vi "DisplayJson.vi"(11 "JSON String In":string="[{\"version\":\"1.0.0\",\"header\":{\"creationDate\":\"2022-06-03T00:00:00\",\"remarks\":\"\",\"serialNumber\":\"98172\",\"productNumber\":\"123021.1804\",\"productType\":\"PAA-9L\",\"pressureType\":2,\"productSeries\":\"9L\",\"compensatedTemperatureRange\":{\"min\":-10.0,\"max\":80.0,\"unit\":4},\"compensatedPressureRange\":{\"min\":0.0,\"max\":0.35,\"unit\":3},\"electricSupply\":{\"magnitude\":1.0,\"unit\":18},\"orderNumber\":9990266,\"orderPosition\":3,\"orderTargetDispatchDate\":\"2022-06-02T00:00:00+00:00\",\"customerName\":\"DemoData Inc.\",\"customerNumber\":12345678,\"customerOrderNumber\":\"Cust-9990266-123\",\"customerReferenceNumber\":\"\",\"customerProductT...") -> ()   [LabVIEW 2017] (continued)
\"unit\":4}}}}}},{\"reference\":\"F_12300_XX_0000098765\",\"environmentTarget\":{\"pressure\":{\"magnitude\":0.11,\"unit\":3},\"temperature\":{\"magnitude\":40.0,\"unit\":4}},\"environment\":{\"pressure\":{\"magnitude\":0.110005,\"unit\":3},\"temperature\":{\"magnitude\":39.7284,\"unit\":4},\"supply\":{\"magnitude\":1.0,\"unit\":18}},\"raw\":{\"signal\":{\"magnitude\":28.847389263,\"unit\":22},\"bridgeResistance\":{\"magnitude\":3661.6768749,\"unit\":28}},\"compensated\":{\"mathematicalModels\":{\"MM0123\":{\"pressure\":{\"output\":{\"magnitude\":0.109977,\"unit\":3},\"error\":{\"magnitude\":-0.0080257298,\"unit\":7}},\"temperature\":{\"output\":{\"magnitude\":39.719,\"unit\":4},\"error\":{\"magnitude\":-0.0094531335,\"unit\":4}}}}}},{\"reference\":\"F_12300_XX_0000098765\",\"environmentTarget\":{\"pressure\":{\"magnitude\":0.19,\"unit\":3},\"temperature\":{\"magnitude\":40.0,\"unit\":4}},\"environment\":{\"pressure\":{\"magnitude\":0.190007,\"unit\":3},\"temperature\":{\"magnitude\":39.7284,\"unit\":4},\"supply\":{\"magnitude\":1.0,\"unit\":18}},\"raw\":{\"signal\":{\"magnitude\":40.361547993,\"unit\":22},\"bridgeResistance\":{\"magnitude\":3657.3317258,\"unit\":28}},\"compensated\":{\"mathematicalModels\":{\"MM0123\":{\"pressure\":{\"output\":{\"magnitude\":0.190005,\"unit\":3},\"error\":{\"magnitude\":-0.00061989229,\"unit\":7}},\"temperature\":{\"output\":{\"magnitude\":39.7158,\"unit\":4},\"error\":{\"magnitude\":-0.012650311,\"unit\":4}}}}}},{\"reference\":\"F_12300_XX_0000098765\",\"environmentTarget\":{\"pressure\":{\"magnitude\":0.27,\"unit\":3},\"temperature\":{\"magnitude\":40.0,\"unit\":4}},\"environment\":{\"pressure\":{\"magnitude\":0.269994,\"unit\":3},\"temperature\":{\"magnitude\":39.7284,\"unit\":4},\"supply\":{\"magnitude\":1.0,\"unit\":18}},\"raw\":{\"signal\":{\"magnitude\":51.835430308,\"unit\":22},\"bridgeResistance\":{\"magnitude\":3653.059498,\"unit\":28}},\"compensated\":{\"mathematicalModels\":{\"MM0123\":{\"pressure\":{\"output\":{\"magnitude\":0.270012,\"unit\":3},\"error\":{\"magnitude\":0.0052035531,\"unit\":7}},\"temperature\":{\"output\":{\"magnitude\":39.7125,\"unit\":4},\"error\":{\"magnitude\":-0.015896776,\"unit\":4}}}}}},{\"reference\":\"F_12300_XX_0000098765\",\"environmentTarget\":{\"pressure\":{\"magnitude\":0.35,\"unit\":3},\"temperature\":{\"magnitude\":40.0,\"unit\":4}},\"environment\":{\"pressure\":{\"magnitude\":0.350005,\"unit\":3},\"temperature\":{\"magnitude\":39.7284,\"unit\":4},\"supply\":{\"magnitude\":1.0,\"unit\":18}},\"raw\":{\"signal\":{\"magnitude\":63.26645716,\"unit\":22},\"bridgeResistance\":{\"magnitude\":3648.8999829,\"unit\":28}},\"compensated\":{\"mathematicalModels\":{\"MM0123\":{\"pressure\":{\"output\":{\"magnitude\":0.349978,\"unit\":3},\"error\":{\"magnitude\":-0.0076198189,\"unit\":7}},\"temperature\":{\"output\":{\"magnitude\":39.7135,\"unit\":4},\"error\":{\"magnitude\":-0.014908129,\"unit\":4}}}}}},{\"reference\":\"F_12300_XX_0000098765\",\"environmentTarget\":{\"pressure\":{\"magnitude\":0.03,\"unit\":3},\"temperature\":{\"magnitude\":60.0,\"unit\":4}},\"environment\":{\"pressure\":{\"magnitude\":0.029994,\"unit\":3},\"temperature\":{\"magnitude\":59.8651,\"unit\":4},\"supply\":{\"magnitude\":1.0,\"unit\":18}},\"raw\":{\"signal\":{\"magnitude\":18.423541771,\"unit\":22},\"bridgeResistance\":{\"magnitude\":3857.3811421,\"unit\":28}},\"compensated\":{\"mathematicalModels\":{\"MM0123\":{\"pressure\":{\"output\":{\"magnitude\":0.0300054,\"unit\":3},\"error\":{\"magnitude\":0.0032489215,\"unit\":7}},\"temperature\":{\"output\":{\"magnitude\":59.9297,\"unit\":4},\"error\":{\"magnitude\":0.064540842,\"unit\":4}}}}}},{\"reference\":\"F_12300_XX_0000098765\",\"environmentTarget\":{\"pressure\":{\"magnitude\":0.11,\"unit\":3},\"temperature\":{\"magnitude\":60.0,\"unit\":4}},\"environment\":{\"pressure\":{\"magnitude\":0.110001,\"unit\":3},\"temperature\":{\"magnitude\":59.8651,\"unit\":4},\"supply\":{\"magnitude\":1.0,\"unit\":18}},\"raw\":{\"signal\":{\"magnitude\":30.058054899,\"unit\":22},\"bridgeResistance\":{\"magnitude\":3852.9241805,\"unit\":28}},\"compensated\":{\"mathematicalModels\":{\"MM0123\":{\"pressure\":{\"output\":{\"magnitude\":0.109972,\"unit\":3},\"error\":{\"magnitude\":-0.0083184018,\"unit\":7}},\"temperature\":{\"output\":{\"magnitude\":59.9321,\"unit\":4},\"error\":{\"magnitude\":0.066957365,\"unit\":4}}}}}},{\"reference\":\"F_12300_XX_0000098765\",\"environmentTarget\":{\"pressure\":{\"magnitude\":0.19,\"unit\":3},\"temperature\":{\"magnitude\":60.0,\"unit\":4}},\"environment\":{\"pressure\":{\"magnitude\":0.189998,\"unit\":3},\"temperature\":{\"magnitude\":59.8651,\"unit\":4},\"supply\":{\"magnitude\":1.0,\"unit\":18}},\"raw\":{\"signal\":{\"magnitude\":41.669413946,\"unit\":22},\"bridgeResistance\":{\"magnitude\":3848.535791,\"unit\":28}},\"compensated\":{\"mathematicalModels\":{\"MM0123\":{\"pressure\":{\"output\":{\"magnitude\":0.190007,\"unit\":3},\"error\":{\"magnitude\":0.0026498924,\"unit\":7}},\"temperature\":{\"output\":{\"magnitude\":59.9347,\"unit\":4},\"error\":{\"magnitude\":0.069571324,\"unit\":4}}}}}},{\"reference\":\"F_12300_XX_0000098765\",\"environmentTarget\":{\"pressure\":{\"magnitude\":0.27,\"unit\":3},\"temperature\":{\"magnitude\":60.0,\"unit\":4}},\"environment\":{\"pressure\":{\"magnitude\":0.270009,\"unit\":3},\"temperature\":{\"magnitude\":59.8651,\"unit\":4},\"supply\":{\"magnitude\":1.0,\"unit\":18}},\"raw\":{\"signal\":{\"magnitude\":53.245645567,\"unit\":22},\"bridgeResistance\":{\"magnitude\":3844.1953821,\"unit\":28}},\"compensated\":{\"mathematicalModels\":{\"MM0123\":{\"pressure\":{\"output\":{\"magnitude\":0.27003,\"unit\":3},\"error\":{\"magnitude\":0.0061415459,\"unit\":7}},\"temperature\":{\"output\":{\"magnitude\":59.935,\"unit\":4},\"error\":{\"magnitude\":0.069824739,\"unit\":4}}}}}},{\"reference\":\"F_12300_XX_0000098765\",\"environmentTarget\":{\"pressure\":{\"magnitude\":0.35,\"unit\":3},\"temperature\":{\"magnitude\":60.0,\"unit\":4}},\"environment\":{\"pressure\":{\"magnitude\":0.349993,\"unit\":3},\"temperature\":{\"magnitude\":59.8651,\"unit\":4},\"supply\":{\"magnitude\":1.0,\"unit\":18}},\"raw\":{\"signal\":{\"magnitude\":64.779425416,\"unit\":22},\"bridgeResistance\":{\"magnitude\":3839.9610565,\"unit\":28}},\"compensated\":{\"mathematicalModels\":{\"MM0123\":{\"pressure\":{\"output\":{\"magnitude\":0.349989,\"unit\":3},\"error\":{\"magnitude\":-0.0015548627,\"unit\":7}},\"temperature\":{\"output\":{\"magnitude\":59.9385,\"unit\":4},\"error\":{\"magnitude\":0.073366412,\"unit\":4}}}}}},{\"reference\":\"F_12300_XX_0000098765\",\"environmentTarget\":{\"pressure\":{\"magnitude\":0.03,\"unit\":3},\"temperature\":{\"magnitude\":80.0,\"unit\":4}},\"environment\":{\"pressure\":{\"magnitude\":0.0299873,\"unit\":3},\"temperature\":{\"magnitude\":79.9513,\"unit\":4},\"supply\":{\"magnitude\":1.0,\"unit\":18}},\"raw\":{\"signal\":{\"magnitude\":19.689044719,\"unit\":22},\"bridgeResistance\":{\"magnitude\":4063.7031412,\"unit\":28}},\"compensated\":{\"mathematicalModels\":{\"MM0123\":{\"pressure\":{\"output\":{\"magnitude\":0.0300057,\"unit\":3},\"error\":{\"magnitude\":0.0052612062,\"unit\":7}},\"temperature\":{\"output\":{\"magnitude\":80.0471,\"unit\":4},\"error\":{\"magnitude\":0.095773122,\"unit\":4}}}}}},{\"reference\":\"F_12300_XX_0000098765\",\"environmentTarget\":{\"pressure\":{\"magnitude\":0.11,\"unit\":3},\"temperature\":{\"magnitude\":80.0,\"unit\":4}},\"environment\":{\"pressure\":{\"magnitude\":0.110002,\"unit\":3},\"temperature\":{\"magnitude\":79.9513,\"unit\":4},\"supply\":{\"magnitude\":1.0,\"unit\":18}},\"raw\":{\"signal\":{\"magnitude\":31.441522599,\"unit\":22},\"bridgeResistance\":{\"magnitude\":4059.1986136,\"unit\":28}},\"compensated\":{\"mathematicalModels\":{\"MM0123\":{\"pressure\":{\"output\":{\"magnitude\":0.109961,\"unit\":3},\"error\":{\"magnitude\":-0.011726953,\"unit\":7}},\"temperature\":{\"output\":{\"magnitude\":80.0515,\"unit\":4},\"error\":{\"magnitude\":0.10020114,\"unit\":4}}}}}},{\"reference\":\"F_12300_XX_0000098765\",\"environmentTarget\":{\"pressure\":{\"magnitude\":0.19,\"unit\":3},\"temperature\":{\"magnitude\":80.0,\"unit\":4}},\"environment\":{\"pressure\":{\"magnitude\":0.189998,\"unit\":3},\"temperature\":{\"magnitude\":79.9513,\"unit\":4},\"supply\":{\"magnitude\":1.0,\"unit\":18}},\"raw\":{\"signal\":{\"magnitude\":43.17950971,\"unit\":22},\"bridgeResistance\":{\"magnitude\":4054.764307,\"unit\":28}},\"compensated\":{\"mathematicalModels\":{\"MM0123\":{\"pressure\":{\"output\":{\"magnitude\":0.190004,\"unit\":3},\"error\":{\"magnitude\":0.0018119172,\"unit\":7}},\"temperature\":{\"output\":{\"magnitude\":80.0589,\"unit\":4},\"error\":{\"magnitude\":0.10748996,\"unit\":4}}}}}},{\"reference\":\"F_12300_XX_0000098765\",\"environmentTarget\":{\"pressure\":{\"magnitude\":0.27,\"unit\":3},\"temperature\":{\"magnitude\":80.0,\"unit\":4}},\"environment\":{\"pressure\":{\"magnitude\":0.270004,\"unit\":3},\"temperature\":{\"magnitude\":79.9513,\"unit\":4},\"supply\":{\"magnitude\":1.0,\"unit\":18}},\"raw\":{\"signal\":{\"magnitude\":54.897603555,\"unit\":22},\"bridgeResistance\":{\"magnitude\":4050.3595337,\"unit\":28}},\"compensated\":{\"mathematicalModels\":{\"MM0123\":{\"pressure\":{\"output\":{\"magnitude\":0.270035,\"unit\":3},\"error\":{\"magnitude\":0.0089730118,\"unit\":7}},\"temperature\":{\"output\":{\"magnitude\":80.0644,\"unit\":4},\"error\":{\"magnitude\":0.11303642,\"unit\":4}}}}}},{\"reference\":\"F_12300_XX_0000098765\",\"environmentTarget\":{\"pressure\":{\"magnitude\":0.35,\"unit\":3},\"temperature\":{\"magnitude\":80.0,\"unit\":4}},\"environment\":{\"pressure\":{\"magnitude\":0.349998,\"unit\":3},\"temperature\":{\"magnitude\":79.9513,\"unit\":4},\"supply\":{\"magnitude\":1.0,\"unit\":18}},\"raw\":{\"signal\":{\"magnitude\":66.555259754,\"unit\":22},\"bridgeResistance\":{\"magnitude\":4046.0193689,\"unit\":28}},\"compensated\":{\"mathematicalModels\":{\"MM0123\":{\"pressure\":{\"output\":{\"magnitude\":0.349982,\"unit\":3},\"error\":{\"magnitude\":-0.0046019641,\"unit\":7}},\"temperature\":{\"output\":{\"magnitude\":80.0708,\"unit\":4},\"error\":{\"magnitude\":0.11943972,\"unit\":4}}}}}}]},{\"version\":\"1.0.0\",\"header\":{\"creationDate\":\"2022-06-03T00:00:00\",\"remarks\":\"\",\"serialNumber\":\"98099\",\"productNumber\":\"123021.1804\",\"productType\":\"PAA-9L\",\"pressureType\":2,\"productSeries\":\"9L\",\"compensatedTemperatureRange\":{\"min\":-10.0,\"max\":80.0,\"unit\":4},\"compensatedPressureRange\":{\"min\":0.0,\"max\":0.35,\"unit\":3},\"electricSupply\":{\"magnitude\":1.0,\"unit\":18},\"orderNumber\":9990266,\"orderPosition\":3,\"orderTargetDispatchDate\":\"2022-06-02T00:00:00+00:00\",\"customerName\":\"DemoData Inc.\",\"customerNumber\":12345678,\"customerOrderNumber\":\"Cust-9990266-123\",\"customerReferenceNumber\":\"\",\"customerProductType\":\"123021-1804 Rev.AA\"},\"compensationMethods\":{\"mathematicalModels\":{\"MM0123\":{\"modelType\":\"MM0123\",\"productNumber\":\"000000.0000\",\"compensatedTemperatureRange\":{\"min\":-10.0,\"max\":80.0,\"unit\":4},\"compensatedPressureRange\":{\"min\":0.0,\"max\":0.35,\"unit\":3},\"electricSupply\":{\"magnitude\":1.0,\"unit\":18},\"parts\":{\"pressure\":{\"inputs\":[\"Sig\",\"R\"],\"output\":\"P\",\"description\":\"P = f(Sig,R)\",\"coefficients\":[[4.38368136989,-0.0044433476217,1.67454376191E-06,-2.82593573136E-10,1.78710396707E-14],[-0.128353766542,0.000136857533338,-5.17224292129E-08,8.68145745915E-12,-5.47259969579E-16],[-0.000197357932491,2.38920701492E-07,-1.05262269893E-10,2.02644369074E-14,-1.44696387706E-18]]},\"temperature\":{\"inputs\":[\"R\",\"Sig\"],\"output\":\"T\",\"description\":\"T = f(R,Sig)\",\"coefficients\":[[-7787.78085303,-8.7799248958,0.0879668432411],[7.61584499705,0.0106523479114,-9.73754475914E-05],[-0.00285848377192,-4.71399016424E-06,4.02054815912E-08],[4.8631349814E-07,9.11830114563E-10,-7.34581256659E-12],[-3.12280024047E-11,-6.53300259126E-14,5.01399203161E-16]]}}}}},\"measurements\":[{\"reference\":\"F_12300_XX_0000098765\",\"environmentTarget\":{\"pressure\":{\"magnitude\":0.03,\"unit\":3},\"temperature\":{\"magnitude\":-10.0,\"unit\":4}},\"environment\":{\"pressure\":{\"magnitude\":0.030006,\"unit\":3},\"temperature\":{\"magnitude\":-10.7286,\"unit\":4},\"supply\":{\"magnitude\":1.0,\"unit\":18}},\"raw\":{\"signal\":{\"magnitude\":15.382051383,\"unit\":22},\"bridgeResistance\":{\"magnitude\":3296.0108973,\"unit\":28}},\"compensated\":{\"mathematicalModels\":{\"MM0123\":{\"pressure\":{\"output\":{\"magnitude\":0.0300125,\"unit\":3},\"error\":{\"magnitude\":0.0018587742,\"unit\":7}},\"temperature\":{\"output\":{\"magnitude\":-10.8353,\"unit\":4},\"error\":{\"magnitude\":-0.10662499,\"unit\":4}}}}}},{\"reference\":\"F_12300_XX_0000098765\",\"environmentTarget\":{\"pressure\":{\"magnitude\":0.11,\"unit\":3},\"temperature\":{\"magnitude\":-10.0,\"unit\":4}},\"environment\":{\"pressure\":{\"magnitude\":0.109993,\"unit\":3},\"temperature\":{\"magnitude\":-10.7286,\"unit\":4},\"supply\":{\"magnitude\":1.0,\"unit\":18}},\"raw\":{\"signal\":{\"magnitude\":26.520570721,\"unit\":22},\"bridgeResistance\":{\"magnitude\":3291.7798573,\"unit\":28}},\"compensated\":{\"mathematicalModels\":{\"MM0123\":{\"pressure\":{\"output\":{\"magnitude\":0.10997,\"unit\":3},\"error\":{\"magnitude\":-0.0066964222,\"unit\":7}},\"temperature\":{\"output\":{\"magnitude\":-10.8379,\"unit\":4},\"error\":{\"magnitude\":-0.10930225,\"unit\":4}}}}}},{\"reference\":\"F_12300_XX_0000098765\",\"environmentTarget\":{\"pressure\":{\"magnitude\":0.19,\"unit\":3},\"temperature\":{\"magnitude\":-10.0,\"unit\":4}},\"environment\":{\"pressure\":{\"magnitude\":0.190007,\"unit\":3},\"temperature\":{\"magnitude\":-10.7286,\"unit\":4},\"supply\":{\"magnitude\":1.0,\"unit\":18}},\"raw\":{\"signal\":{\"magnitude\":37.627474048,\"unit\":22},\"bridgeResistance\":{\"magnitude\":3287.6709403,\"unit\":28}},\"compensated\":{\"mathematicalModels\":{\"MM0123\":{\"pressure\":{\"output\":{\"magnitude\":0.190014,\"unit\":3},\"error\":{\"magnitude\":0.0020766896,\"unit\":7}},\"temperature\":{\"output\":{\"magnitude\":-10.8364,\"unit\":4},\"error\":{\"magnitude\":-0.10780221,\"unit\":4}}}}}},{\"reference\":\"F_12300_XX_0000098765\",\"environmentTarget\":{\"pressure\":{\"magnitude\":0.27,\"unit\":3},\"temperature\":{\"magnitude\":-10.0,\"unit\":4}},\"environment\":{\"pressure\":{\"magnitude\":0.270004,\"unit\":3},\"temperature\":{\"magnitude\":-10.7286,\"unit\":4},\"supply\":{\"magnitude\":1.0,\"unit\":18}},\"raw\":{\"signal\":{\"magnitude\":48.686180416,\"unit\":22},\"bridgeResistance\":{\"magnitude\":3283.6800431,\"unit\":28}},\"compensated\":{\"mathematicalModels\":{\"MM0123\":{\"pressure\":{\"output\":{\"magnitude\":0.270029,\"unit\":3},\"error\":{\"magnitude\":0.0071670841,\"unit\":7}},\"temperature\":{\"output\":{\"magnitude\":-10.8323,\"unit\":4},\"error\":{\"magnitude\":-0.10365432,\"unit\":4}}}}}},{\"reference\":\"F_12300_XX_0000098765\",\"environmentTarget\":{\"pressure\":{\"magnitude\":0.35,\"unit\":3},\"temperature\":{\"magnitude\":-10.0,\"unit\":4}},\"environment\":{\"pressure\":{\"magnitude\":0.349999,\"unit\":3},\"temperature\":{\"magnitude\":-10.7286,\"unit\":4},\"supply\":{\"magnitude\":1.0,\"unit\":18}},\"raw\":{\"signal\":{\"magnitude\":59.693656638,\"unit\":22},\"bridgeResistance\":{\"magnitude\":3279.7180932,\"unit\":28}},\"compensated\":{\"mathematicalModels\":{\"MM0123\":{\"pressure\":{\"output\":{\"magnitude\":0.349995,\"unit\":3},\"error\":{\"magnitude\":-0.0010161733,\"unit\":7}},\"temperature\":{\"output\":{\"magnitude\":-10.8389,\"unit\":4},\"error\":{\"magnitude\":-0.11022499,\"unit\":4}}}}}},{\"reference\":\"F_12300_XX_0000098765\",\"environmentTarget\":{\"pressure\":{\"magnitude\":0.03,\"unit\":3},\"temperature\":{\"magnitude\":0.0,\"unit\":4}},\"environment\":{\"pressure\":{\"magnitude\":0.0299976,\"unit\":3},\"temperature\":{\"magnitude\":-0.629962,\"unit\":4},\"supply\":{\"magnitude\":1.0,\"unit\":18}},\"raw\":{\"signal\":{\"magnitude\":15.845157878,\"unit\":22},\"bridgeResistance\":{\"magnitude\":3366.4591239,\"unit\":28}},\"compensated\":{\"mathematicalModels\":{\"MM0123\":{\"pressure\":{\"output\":{\"magnitude\":0.030013,\"unit\":3},\"error\":{\"magnitude\":0.0043993953,\"unit\":7}},\"temperature\":{\"output\":{\"magnitude\":-0.744098,\"unit\":4},\"error\":{\"magnitude\":-0.11413616,\"unit\":4}}}}}},{\"reference\":\"F_12300_XX_0000098765\",\"environmentTarget\":{\"pressure\":{\"magnitude\":0.11,\"unit\":3},\"temperature\":{\"magnitude\":0.0,\"unit\":4}},\"environment\":{\"pressure\":{\"magnitude\":0.110002,\"unit\":3},\"temperature\":{\"magnitude\":-0.629962,\"unit\":4},\"supply\":{\"magnitude\":1.0,\"unit\":18}},\"raw\":{\"signal\":{\"magnitude\":26.952305705,\"unit\":22},\"bridgeResistance\":{\"magnitude\":3362.194976,\"unit\":28}},\"compensated\":{\"mathematicalModels\":{\"MM0123\":{\"pressure\":{\"output\":{\"magnitude\":0.109979,\"unit\":3},\"error\":{\"magnitude\":-0.0065740425,\"unit\":7}},\"temperature\":{\"output\":{\"magnitude\":-0.750974,\"unit\":4},\"error\":{\"magnitude\":-0.12101261,\"unit\":4}}}}}},{\"reference\":\"F_12300_XX_0000098765\",\"environmentTarget\":{\"pressure\":{\"magnitude\":0.19,\"unit\":3},\"temperature\":{\"magnitude\":0.0,\"unit\":4}},\"environment\":{\"pressure\":{\"magnitude\":0.190001,\"unit\":3},\"temperature\":{\"magnitude\":-0.629962,\"unit\":4},\"supply\":{\"magnitude\":1.0,\"unit\":18}},\"raw\":{\"signal\":{\"magnitude\":38.02508102,\"unit\":22},\"bridgeResistance\":{\"magnitude\":3358.0870163,\"unit\":28}},\"compensated\":{\"mathematicalModels\":{\"MM0123\":{\"pressure\":{\"output\":{\"magnitude\":0.189997,\"unit\":3},\"error\":{\"magnitude\":-0.0012005568,\"unit\":7}},\"temperature\":{\"output\":{\"magnitude\":-0.749134,\"unit\":4},\"error\":{\"magnitude\":-0.11917182,\"unit\":4}}}}}},{\"reference\":\"F_12300_XX_0000098765\",\"environmentTarget\":{\"pressure\":{\"magnitude\":0.27,\"unit\":3},\"temperature\":{\"magnitude\":0.0,\"unit\":4}},\"environment\":{\"pressure\":{\"magnitude\":0.269998,\"unit\":3},\"temperature\":{\"magnitude\":-0.629962,\"unit\":4},\"supply\":{\"magnitude\":1.0,\"unit\":18}},\"raw\":{\"signal\":{\"magnitude\":49.054195601,\"unit\":22},\"bridgeResistance\":{\"magnitude\":3354.0154962,\"unit\":28}},\"compensated\":{\"mathematicalModels\":{\"MM0123\":{\"pressure\":{\"output\":{\"magnitude\":0.270005,\"unit\":3},\"error\":{\"magnitude\":0.0021281086,\"unit\":7}},\"temperature\":{\"output\":{\"magnitude\":-0.755647,\"unit\":4},\"error\":{\"magnitude\":-0.12568503,\"unit\":4}}}}}},{\"reference\":\"F_12300_XX_0000098765\",\"environmentTarget\":{\"pressure\":{\"magnitude\":0.35,\"unit\":3},\"temperature\":{\"magnitude\":0.0,\"unit\":4}},\"environment\":{\"pressure\":{\"magnitude\":0.350003,\"unit\":3},\"temperature\":{\"magnitude\":-0.629962,\"unit\":4},\"supply\":{\"magnitude\":1.0,\"unit\":18}},\"raw\":{\"signal\":{\"magnitude\":60.036396279,\"unit\":22},\"bridgeResistance\":{\"magnitude\":3350.0808009,\"unit\":28}},\"compensated\":{\"mathematicalModels\":{\"MM0123\":{\"pressure\":{\"output\":{\"magnitude\":0.349977,\"unit\":3},\"error\":{\"magnitude\":-0.0073024629,\"unit\":7}},\"temperature\":{\"output\":{\"magnitude\":-0.756931,\"unit\":4},\"error\":{\"magnitude\":-0.12696962,\"unit\":4}}}}}},{\"reference\":\"F_12300_XX_0000098765\",\"environmentTarget\":{\"pressure\":{\"magnitude\":0.03,\"unit\":3},\"temperature\":{\"magnitude\":20.0,\"unit\":4}},\"environment\":{\"pressure\":{\"magnitude\":0.0300008,\"unit\":3},\"temperature\":{\"magnitude\":19.5509,\"unit\":4},\"supply\":{\"magnitude\":1.0,\"unit\":18}},\"raw\":{\"signal\":{\"magnitude\":16.806320119,\"unit\":22},\"bridgeResistance\":{\"magnitude\":3524.4564975,\"unit\":28}},\"compensated\":{\"mathematicalModels\":{\"MM0123\":{\"pressure\":{\"output\":{\"magnitude\":0.0300083,\"unit\":3},\"error\":{\"magnitude\":0.0021344829,\"unit\":7}},\"temperature\":{\"output\":{\"magnitude\":19.5478,\"unit\":4},\"error\":{\"magnitude\":-0.0030800173,\"unit\":4}}}}}},{\"reference\":\"F_12300_XX_0000098765\",\"environmentTarget\":{\"pressure\":{\"magnitude\":0.11,\"unit\":3},\"temperature\":{\"magnitude\":20.0,\"unit\":4}},\"environment\":{\"pressure\":{\"magnitude\":0.110003,\"unit\":3},\"temperature\":{\"magnitude\":19.5509,\"unit\":4},\"supply\":{\"magnitude\":1.0,\"unit\":18}},\"raw\":{\"signal\":{\"magnitude\":27.904099212,\"unit\":22},\"bridgeResistance\":{\"magnitude\":3520.2315408,\"unit\":28}},\"compensated\":{\"mathematicalModels\":{\"MM0123\":{\"pressure\":{\"output\":{\"magnitude\":0.109977,\"unit\":3},\"error\":{\"magnitude\":-0.0073978405,\"unit\":7}},\"temperature\":{\"output\":{\"magnitude\":19.5451,\"unit\":4},\"error\":{\"magnitude\":-0.0057708156,\"unit\":4}}}}}},{\"reference\":\"F_12300_XX_0000098765\",\"environmentTarget\":{\"pressure\":{\"magnitude\":0.19,\"unit\":3},\"temperature\":{\"magnitude\":20.0,\"unit\":4}},\"environment\":{\"pressure\":{\"magnitude\":0.189994,\"unit\":3},\"temperature\":{\"magnitude\":19.5509,\"unit\":4},\"supply\":{\"magnitude\":1.0,\"unit\":18}},\"raw\":{\"signal\":{\"magnitude\":38.97306418,\"unit\":22},\"bridgeResistance\":{\"magnitude\":3516.1095813,\"unit\":28}},\"compensated\":{\"mathematicalModels\":{\"MM0123\":{\"pressure\":{\"output\":{\"magnitude\":0.190009,\"unit\":3},\"error\":{\"magnitude\":0.0043644814,\"unit\":7}},\"temperature\":{\"output\":{\"magnitude\":19.5455,\"unit\":4},\"error\":{\"magnitude\":-0.0053955053,\"unit\":4}}}}}},{\"reference\":\"F_12300_XX_0000098765\",\"environmentTarget\":{\"pressure\":{\"magnitude\":0.27,\"unit\":3},\"temperature\":{\"magnitude\":20.0,\"unit\":4}},\"environment\":{\"pressure\":{\"magnitude\":0.269991,\"unit\":3},\"temperature\":{\"magnitude\":19.5509,\"unit\":4},\"supply\":{\"magnitude\":1.0,\"unit\":18}},\"raw\":{\"signal\":{\"magnitude\":50.000947506,\"unit\":22},\"bridgeResistance\":{\"magnitude\":3512.0209561,\"unit\":28}},\"compensated\":{\"mathematicalModels\":{\"MM0123\":{\"pressure\":{\"output\":{\"magnitude\":0.27002,\"unit\":3},\"error\":{\"magnitude\":0.0082112904,\"unit\":7}},\"temperature\":{\"output\":{\"magnitude\":19.5399,\"unit\":4},\"error\":{\"magnitude\":-0.011025876,\"unit\":4}}}}}},{\"reference\":\"F_12300_XX_0000098765\",\"environmentTarget\":{\"pressure\":{\"magnitude\":0.35,\"unit\":3},\"temperature\":{\"magnitude\":20.0,\"unit\":4}},\"environment\":{\"pressure\":{\"magnitude\":0.350008,\"unit\":3},\"temperature\":{\"magnitude\":19.5509,\"unit\":4},\"supply\":{\"magnitude\":1.0,\"unit\":18}},\"raw\":{\"signal\":{\"magnitude\":60.989084338,\"unit\":22},\"bridgeResistance\":{\"magnitude\":3508.0484262,\"unit\":28}},\"compensated\":{\"mathematicalModels\":{\"MM0123\":{\"pressure\":{\"output\":{\"magnitude\":0.350014,\"unit\":3},\"error\":{\"magnitude\":0.0017915657,\"unit\":7}},\"temperature\":{\"output\":{\"magnitude\":19.5381,\"unit\":4},\"error\":{\"magnitude\":-0.012809606,\"unit\":4}}}}}},{\"reference\":\"F_12300_XX_0000098765\",\"environmentTarget\":{\"pressure\":{\"magnitude\":0.03,\"unit\":3},\"temperature\":{\"magnitude\":40.0,\"unit\":4}},\"environment\":{\"pressure\":{\"magnitude\":0.0300067,\"unit\":3},\"temperature\":{\"magnitude\":39.7284,\"unit\":4},\"supply\":{\"magnitude\":1.0,\"unit\":18}},\"raw\":{\"signal\":{\"magnitude\":17.833834451,\"unit\":22},\"bridgeResistance\":{\"magnitude\":3701.5170718,\"unit\":28}},\"compensated\":{\"mathematicalModels\":{\"MM0123\":{\"pressure\":{\"output\":{\"magnitude\":0.0300226,\"unit\":3},\"error\":{\"magnitude\":0.0045412863,\"unit\":7}},\"temperature\":{\"output\":{\"magnitude\":39.7199,\"unit\":4},\"error\":{\"magnitude\":-0.0085106078,\"unit\":4}}}}}},{\"reference\":\"F_12300_XX_0000098765\",\"environmentTarget\":{\"pressure\":{\"magnitude\":0.11,\"unit\":3},\"temperature\":{\"magnitude\":40.0,\"unit\":4}},\"environment\":{\"pressure\":{\"magnitude\":0.110003,\"unit\":3},\"temperature\":{\"magnitude\":39.7284,\"unit\":4},\"supply\":{\"magnitude\":1.0,\"unit\":18}},\"raw\":{\"signal\":{\"magnitude\":28.980195911,\"unit\":22},\"bridgeResistance\":{\"magnitude\":3697.2936565,\"unit\":28}},\"compensated\":{\"mathematicalModels\":{\"MM0123\":{\"pressure\":{\"output\":{\"magnitude\":0.109976,\"unit\":3},\"error\":{\"magnitude\":-0.0077360363,\"unit\":7}},\"temperature\":{\"output\":{\"magnitude\":39.7196,\"unit\":4},\"error\":{\"magnitude\":-0.0089684403,\"unit\":4}}}}}},{\"reference\":\"F_12300_XX_0000098765\",\"environmentTarget\":{\"pressure\":{\"magnitude\":0.19,\"unit\":3},\"temperature\":{\"magnitude\":40.0,\"unit\":4}},\"environment\":{\"pressure\":{\"magnitude\":0.190004,\"unit\":3},\"temperature\":{\"magnitude\":39.7284,\"unit\":4},\"supply\":{\"magnitude\":1.0,\"unit\":18}},\"raw\":{\"signal\":{\"magnitude\":40.102759224,\"unit\":22},\"bridgeResistance\":{\"magnitude\":3693.0940203,\"unit\":28}},\"compensated\":{\"mathematicalModels\":{\"MM0123\":{\"pressure\":{\"output\":{\"magnitude\":0.190002,\"unit\":3},\"error\":{\"magnitude\":-0.00064045103,\"unit\":7}},\"temperature\":{\"output\":{\"magnitude\":39.7149,\"unit\":4},\"error\":{\"magnitude\":-0.013507331,\"unit\":4}}}}}},{\"reference\":\"F_12300_XX_0000098765\",\"environmentTarget\":{\"pressure\":{\"magnitude\":0.27,\"unit\":3},\"temperature\":{\"magnitude\":40.0,\"unit\":4}},\"environment\":{\"pressure\":{\"magnitude\":0.269991,\"unit\":3},\"temperature\":{\"magnitude\":39.7284,\"unit\":4},\"supply\":{\"magnitude\":1.0,\"unit\":18}},\"raw\":{\"signal\":{\"magnitude\":51.189626064,\"unit\":22},\"bridgeResistance\":{\"magnitude\":3689.9929529,\"unit\":28}},\"compensated\":{\"mathematicalModels\":{\"MM0123\":{\"pressure\":{\"output\":{\"magnitude\":0.270004,\"unit\":3},\"error\":{\"magnitude\":0.0037832258,\"unit\":7}},\"temperature\":{\"output\":{\"magnitude\":39.7135,\"unit\":4},\"error\":{\"magnitude\":-0.014897162,\"unit\":4}}}}}},{\"reference\":\"F_12300_XX_0000098765\",\"environmentTarget\":{\"pressure\":{\"magnitude\":0.35,\"unit\":3},\"temperature\":{\"magnitude\":40.0,\"unit\":4}},\"environment\":{\"pressure\":{\"magnitude\":0.349999,\"unit\":3},\"temperature\":{\"magnitude\":39.7284,\"unit\":4},\"supply\":{\"magnitude\":1.0,\"unit\":18}},\"raw\":{\"signal\":{\"magnitude\":62.236860878,\"unit\":22},\"bridgeResistance\":{\"magnitude\":3684.974664,\"unit\":28}},\"compensated\":{\"mathematicalModels\":{\"MM0123\":{\"pressure\":{\"output\":{\"magnitude\":0.349977,\"unit\":3},\"error\":{\"magnitude\":-0.0063524258,\"unit\":7}},\"temperature\":{\"output\":{\"magnitude\":39.7136,\"unit\":4},\"error\":{\"magnitude\":-0.014833646,\"unit\":4}}}}}},{\"reference\":\"F_12300_XX_0000098765\",\"environmentTarget\":{\"pressure\":{\"magnitude\":0.03,\"unit\":3},\"temperature\":{\"magnitude\":60.0,\"unit\":4}},\"environment\":{\"pressure\":{\"magnitude\":0.0299965,\"unit\":3},\"temperature\":{\"magnitude\":59.8651,\"unit\":4},\"supply\":{\"magnitude\":1.0,\"unit\":18}},\"raw\":{\"signal\":{\"magnitude\":18.961035266,\"unit\":22},\"bridgeResistance\":{\"magnitude\":3894.9657238,\"unit\":28}},\"compensated\":{\"mathematicalModels\":{\"MM0123\":{\"pressure\":{\"output\":{\"magnitude\":0.030008,\"unit\":3},\"error\":{\"magnitude\":0.003299773,\"unit\":7}},\"temperature\":{\"output\":{\"magnitude\":59.9297,\"unit\":4},\"error\":{\"magnitude\":0.064552833,\"unit\":4}}}}}},{\"reference\":\"F_12300_XX_0000098765\",\"environmentTarget\":{\"pressure\":{\"magnitude\":0.11,\"unit\":3},\"temperature\":{\"magnitude\":60.0,\"unit\":4}},\"environment\":{\"pressure\":{\"magnitude\":0.110001,\"unit\":3},\"temperature\":{\"magnitude\":59.8651,\"unit\":4},\"supply\":{\"magnitude\":1.0,\"unit\":18}},\"raw\":{\"signal\":{\"magnitude\":30.197358349,\"unit\":22},\"bridgeResistance\":{\"magnitude\":3890.6765324,\"unit\":28}},\"compensated\":{\"mathematicalModels\":{\"MM0123\":{\"pressure\":{\"output\":{\"magnitude\":0.109974,\"unit\":3},\"error\":{\"magnitude\":-0.0078152898,\"unit\":7}},\"temperature\":{\"output\":{\"magnitude\":59.9317,\"unit\":4},\"error\":{\"magnitude\":0.066609874,\"unit\":4}}}}}},{\"reference\":\"F_12300_XX_0000098765\",\"environmentTarget\":{\"pressure\":{\"magnitude\":0.19,\"unit\":3},\"temperature\":{\"magnitude\":60.0,\"unit\":4}},\"environment\":{\"pressure\":{\"magnitude\":0.190002,\"unit\":3},\"temperature\":{\"magnitude\":59.8651,\"unit\":4},\"supply\":{\"magnitude\":1.0,\"unit\":18}},\"raw\":{\"signal\":{\"magnitude\":41.413877452,\"unit\":22},\"bridgeResistance\":{\"magnitude\":3896.4601228,\"unit\":28}},\"compensated\":{\"mathematicalModels\":{\"MM0123\":{\"pressure\":{\"output\":{\"magnitude\":0.190009,\"unit\":3},\"error\":{\"magnitude\":0.0020187471,\"unit\":7}},\"temperature\":{\"output\":{\"magnitude\":59.935,\"unit\":4},\"error\":{\"magnitude\":0.069867909,\"unit\":4}}}}}},{\"reference\":\"F_12300_XX_0000098765\",\"environmentTarget\":{\"pressure\":{\"magnitude\":0.27,\"unit\":3},\"temperature\":{\"magnitude\":60.0,\"unit\":4}},\"environment\":{\"pressure\":{\"magnitude\":0.270004,\"unit\":3},\"temperature\":{\"magnitude\":59.8651,\"unit\":4},\"supply\":{\"magnitude\":1.0,\"unit\":18}},\"raw\":{\"signal\":{\"magnitude\":52.598121445,\"unit\":22},\"bridgeResistance\":{\"magnitude\":3892.2685447,\"unit\":28}},\"compensated\":{\"mathematicalModels\":{\"MM0123\":{\"pressure\":{\"output\":{\"magnitude\":0.270028,\"unit\":3},\"error\":{\"magnitude\":0.0069317542,\"unit\":7}},\"temperature\":{\"output\":{\"magnitude\":59.9342,\"unit\":4},\"error\":{\"magnitude\":0.069045083,\"unit\":4}}}}}},{\"reference\":\"F_12300_XX_0000098765\",\"environmentTarget\":{\"pressure\":{\"magnitude\":0.35,\"unit\":3},\"temperature\":{\"magnitude\":60.0,\"unit\":4}},\"environment\":{\"pressure\":{\"magnitude\":0.349995,\"unit\":3},\"temperature\":{\"magnitude\":59.8651,\"unit\":4},\"supply\":{\"magnitude\":1.0,\"unit\":18}},\"raw\":{\"signal\":{\"magnitude\":63.744638356,\"unit\":22},\"bridgeResistance\":{\"magnitude\":3878.1913733,\"unit\":28}},\"compensated\":{\"mathematicalModels\":{\"MM0123\":{\"pressure\":{\"output\":{\"magnitude\":0.349987,\"unit\":3},\"error\":{\"magnitude\":-0.0021959248,\"unit\":7}},\"temperature\":{\"output\":{\"magnitude\":59.9381,\"unit\":4},\"error\":{\"magnitude\":0.072975962,\"unit\":4}}}}}},{\"reference\":\"F_12300_XX_0000098765\",\"environmentTarget\":{\"pressure\":{\"magnitude\":0.03,\"unit\":3},\"temperature\":{\"magnitude\":80.0,\"unit\":4}},\"environment\":{\"pressure\":{\"magnitude\":0.0299926,\"unit\":3},\"temperature\":{\"magnitude\":79.9513,\"unit\":4},\"supply\":{\"magnitude\":1.0,\"unit\":18}},\"raw\":{\"signal\":{\"magnitude\":20.229826455,\"unit\":22},\"bridgeResistance\":{\"magnitude\":4103.5739894,\"unit\":28}},\"compensated\":{\"mathematicalModels\":{\"MM0123\":{\"pressure\":{\"output\":{\"magnitude\":0.0300062,\"unit\":3},\"error\":{\"magnitude\":0.0038785897,\"unit\":7}},\"temperature\":{\"output\":{\"magnitude\":80.0466,\"unit\":4},\"error\":{\"magnitude\":0.095250938,\"unit\":4}}}}}},{\"reference\":\"F_12300_XX_0000098765\",\"environmentTarget\":{\"pressure\":{\"magnitude\":0.11,\"unit\":3},\"temperature\":{\"magnitude\":80.0,\"unit\":4}},\"environment\":{\"pressure\":{\"magnitude\":0.109996,\"unit\":3},\"temperature\":{\"magnitude\":79.9513,\"unit\":4},\"supply\":{\"magnitude\":1.0,\"unit\":18}},\"raw\":{\"signal\":{\"magnitude\":31.580347145,\"unit\":22},\"bridgeResistance\":{\"magnitude\":4099.2357604,\"unit\":28}},\"compensated\":{\"mathematicalModels\":{\"MM0123\":{\"pressure\":{\"output\":{\"magnitude\":0.109965,\"unit\":3},\"error\":{\"magnitude\":-0.0089056769,\"unit\":7}},\"temperature\":{\"output\":{\"magnitude\":80.0506,\"unit\":4},\"error\":{\"magnitude\":0.099228491,\"unit\":4}}}}}},{\"reference\":\"F_12300_XX_0000098765\",\"environmentTarget\":{\"pressure\":{\"magnitude\":0.19,\"unit\":3},\"temperature\":{\"magnitude\":80.0,\"unit\":4}},\"environment\":{\"pressure\":{\"magnitude\":0.19,\"unit\":3},\"temperature\":{\"magnitude\":79.9513,\"unit\":4},\"supply\":{\"magnitude\":1.0,\"unit\":18}},\"raw\":{\"signal\":{\"magnitude\":42.917977519,\"unit\":22},\"bridgeResistance\":{\"magnitude\":4094.9684649,\"unit\":28}},\"compensated\":{\"mathematicalModels\":{\"MM0123\":{\"pressure\":{\"output\":{\"magnitude\":0.190005,\"unit\":3},\"error\":{\"magnitude\":0.0012893248,\"unit\":7}},\"temperature\":{\"output\":{\"magnitude\":80.0578,\"unit\":4},\"error\":{\"magnitude\":0.10641535,\"unit\":4}}}}}},{\"reference\":\"F_12300_XX_0000098765\",\"environmentTarget\":{\"pressure\":{\"magnitude\":0.27,\"unit\":3},\"temperature\":{\"magnitude\":80.0,\"unit\":4}},\"environment\":{\"pressure\":{\"magnitude\":0.270005,\"unit\":3},\"temperature\":{\"magnitude\":79.9513,\"unit\":4},\"supply\":{\"magnitude\":1.0,\"unit\":18}},\"raw\":{\"signal\":{\"magnitude\":54.228411217,\"unit\":22},\"bridgeResistance\":{\"magnitude\":4090.7227383,\"unit\":28}},\"compensated\":{\"mathematicalModels\":{\"MM0123\":{\"pressure\":{\"output\":{\"magnitude\":0.270029,\"unit\":3},\"error\":{\"magnitude\":0.0068921791,\"unit\":7}},\"temperature\":{\"output\":{\"magnitude\":80.0628,\"unit\":4},\"error\":{\"magnitude\":0.11248648,\"unit\":4}}}}}},{\"reference\":\"F_12300_XX_0000098765\",\"environmentTarget\":{\"pressure\":{\"magnitude\":0.35,\"unit\":3},\"temperature\":{\"magnitude\":80.0,\"unit\":4}},\"environment\":{\"pressure\":{\"magnitude\":0.35,\"unit\":3},\"temperature\":{\"magnitude\":79.9513,\"unit\":4},\"supply\":{\"magnitude\":1.0,\"unit\":18}},\"raw\":{\"signal\":{\"magnitude\":65.504630357,\"unit\":22},\"bridgeResistance\":{\"magnitude\":4086.5380461,\"unit\":28}},\"compensated\":{\"mathematicalModels\":{\"MM0123\":{\"pressure\":{\"output\":{\"magnitude\":0.349989,\"unit\":3},\"error\":{\"magnitude\":-0.0033144596,\"unit\":7}},\"temperature\":{\"output\":{\"magnitude\":80.0689,\"unit\":4},\"error\":{\"magnitude\":0.11751968,\"unit\":4}}}}}}]},{\"version\":\"1.0.0\",\"header\":{\"creationDate\":\"2022-06-03T00:00:00\",\"remarks\":\"\",\"serialNumber\":\"98091\",\"productNumber\":\"123021.1804\",\"productType\":\"PAA-9L\",\"pressureType\":2,\"productSeries\":\"9L\",\"compensatedTemperatureRange\":{\"min\":-10.0,\"max\":80.0,\"unit\":4},\"compensatedPressureRange\":{\"min\":0.0,\"max\":0.35,\"unit\":3},\"electricSupply\":{\"magnitude\":1.0,\"unit\":18},\"orderNumber\":9990266,\"orderPosition\":3,\"orderTargetDispatchDate\":\"2022-06-02T00:00:00+00:00\",\"customerName\":\"DemoData Inc.\",\"customerNumber\":12345678,\"customerOrderNumber\":\"Cust-9990266-123\",\"customerReferenceNumber\":\"\",\"customerProductType\":\"123021-1804 Rev.AA\"},\"compensationMethods\":{\"mathematicalModels\":{\"MM0123\":{\"modelType\":\"MM0123\",\"productNumber\":\"000000.0000\",\"compensatedTemperatureRange\":{\"min\":-10.0,\"max\":80.0,\"unit\":4},\"compensatedPressureRange\":{\"min\":0.0,\"max\":0.35,\"unit\":3},\"electricSupply\":{\"magnitude\":1.0,\"unit\":18},\"parts\":{\"pressure\":{\"inputs\":[\"Sig\",\"R\"],\"output\":\"P\",\"description\":\"P = f(Sig,R)\",\"coefficients\":[[4.95454369386,-0.00509348764714,1.9452606504E-06,-3.3233240917E-10,2.12676620418E-14],[-0.198614166283,0.000215308655021,-8.4318245041E-08,1.46789166733E-11,-9.59749626915E-16],[0.000578750204434,-6.10969838785E-07,2.42979713656E-10,-4.30154975687E-14,2.85557553484E-18]]},\"temperature\":{\"inputs\":[\"R\",\"Sig\"],\"output\":\"T\",\"description\":\"T = f(R,Sig)\",\"coefficients\":[[-7649.03316349,-16.8444396952,0.170857740122],[7.54365756153,0.0196472748786,-0.000189425101321],[-0.00285675980662,-8.4735210919E-06,7.84412085529E-08],[4.90576357124E-07,1.60943908994E-09,-1.43868944661E-11],[-3.18014839539E-11,-1.13807272441E-13,9.86422086573E-16]]}}}}},\"measurements\":[{\"reference\":\"F_12300_XX_0000098765\",\"environmentTarget\":{\"pressure\":{\"magnitude\":0.03,\"unit\":3},\"temperature\":{\"magnitude\":-10.0,\"unit\":4}},\"environment\":{\"pressure\":{\"magnitude\":0.0300056,\"unit\":3},\"temperature\":{\"magnitude\":-10.7286,\"unit\":4},\"supply\":{\"magnitude\":1.0,\"unit\":18}},\"raw\":{\"signal\":{\"magnitude\":16.121143048,\"unit\":22},\"bridgeResistance\":{\"magnitude\":3265.2678464,\"unit\":28}},\"compensated\":{\"mathematicalModels\":{\"MM0123\":{\"pressure\":{\"output\":{\"magnitude\":0.0300113,\"unit\":3},\"error\":{\"magnitude\":0.0016247293,\"unit\":7}},\"temperature\":{\"output\":{\"magnitude\":-10.8348,\"unit\":4},\"error\":{\"magnitude\":-0.10616952,\"unit\":4}}}}}},{\"reference\":\"F_12300_XX_0000098765\",\"environmentTarget\":{\"pressure\":{\"magnitude\":0.11,\"unit\":3},\"temperature\":{\"magnitude\":-10.0,\"unit\":4}},\"environment\":{\"pressure\":{\"magnitude\":0.109994,\"unit\":3},\"temperature\":{\"magnitude\":-10.7286,\"unit\":4},\"supply\":{\"magnitude\":1.0,\"unit\":18}},\"raw\":{\"signal\":{\"magnitude\":26.872052787,\"unit\":22},\"bridgeResistance\":{\"magnitude\":3261.2090129,\"unit\":28}},\"compensated\":{\"mathematicalModels\":{\"MM0123\":{\"pressure\":{\"output\":{\"magnitude\":0.109969,\"unit\":3},\"error\":{\"magnitude\":-0.0071462632,\"unit\":7}},\"temperature\":{\"output\":{\"magnitude\":-10.8381,\"unit\":4},\"error\":{\"magnitude\":-0.10943727,\"unit\":4}}}}}},{\"reference\":\"F_12300_XX_0000098765\",\"environmentTarget\":{\"pressure\":{\"magnitude\":0.19,\"unit\":3},\"temperature\":{\"magnitude\":-10.0,\"unit\":4}},\"environment\":{\"pressure\":{\"magnitude\":0.190007,\"unit\":3},\"temperature\":{\"magnitude\":-10.7286,\"unit\":4},\"supply\":{\"magnitude\":1.0,\"unit\":18}},\"raw\":{\"signal\":{\"magnitude\":37.593551332,\"unit\":22},\"bridgeResistance\":{\"magnitude\":3257.2770294,\"unit\":28}},\"compensated\":{\"mathematicalModels\":{\"MM0123\":{\"pressure\":{\"output\":{\"magnitude\":0.19001,\"unit\":3},\"error\":{\"magnitude\":0.00084189031,\"unit\":7}},\"temperature\":{\"output\":{\"magnitude\":-10.8361,\"unit\":4},\"error\":{\"magnitude\":-0.10746417,\"unit\":4}}}}}},{\"reference\":\"F_12300_XX_0000098765\",\"environmentTarget\":{\"pressure\":{\"magnitude\":0.27,\"unit\":3},\"temperature\":{\"magnitude\":-10.0,\"unit\":4}},\"environment\":{\"pressure\":{\"magnitude\":0.270004,\"unit\":3},\"temperature\":{\"magnitude\":-10.7286,\"unit\":4},\"supply\":{\"magnitude\":1.0,\"unit\":18}},\"raw\":{\"signal\":{\"magnitude\":48.2711502,\"unit\":22},\"bridgeResistance\":{\"magnitude\":3253.4652947,\"unit\":28}},\"compensated\":{\"mathematicalModels\":{\"MM0123\":{\"pressure\":{\"output\":{\"magnitude\":0.27003,\"unit\":3},\"error\":{\"magnitude\":0.0073605207,\"unit\":7}},\"temperature\":{\"output\":{\"magnitude\":-10.8306,\"unit\":4},\"error\":{\"magnitude\":-0.10191956,\"unit\":4}}}}}},{\"reference\":\"F_12300_XX_0000098765\",\"environmentTarget\":{\"pressure\":{\"magnitude\":0.35,\"unit\":3},\"temperature\":{\"magnitude\":-10.0,\"unit\":4}},\"environment\":{\"pressure\":{\"magnitude\":0.350007,\"unit\":3},\"temperature\":{\"magnitude\":-10.7286,\"unit\":4},\"supply\":{\"magnitude\":1.0,\"unit\":18}},\"raw\":{\"signal\":{\"magnitude\":58.900635465,\"unit\":22},\"bridgeResistance\":{\"magnitude\":3249.665179,\"unit\":28}},\"compensated\":{\"mathematicalModels\":{\"MM0123\":{\"pressure\":{\"output\":{\"magnitude\":0.350003,\"unit\":3},\"error\":{\"magnitude\":-0.0012028983,\"unit\":7}},\"temperature\":{\"output\":{\"magnitude\":-10.8378,\"unit\":4},\"error\":{\"magnitude\":-0.10912855,\"unit\":4}}}}}},{\"reference\":\"F_12300_XX_0000098765\",\"environmentTarget\":{\"pressure\":{\"magnitude\":0.03,\"unit\":3},\"temperature\":{\"magnitude\":0.0,\"unit\":4}},\"environment\":{\"pressure\":{\"magnitude\":0.0299956,\"unit\":3},\"temperature\":{\"magnitude\":-0.629962,\"unit\":4},\"supply\":{\"magnitude\":1.0,\"unit\":18}},\"raw\":{\"signal\":{\"magnitude\":16.581912009,\"unit\":22},\"bridgeResistance\":{\"magnitude\":3335.2008701,\"unit\":28}},\"compensated\":{\"mathematicalModels\":{\"MM0123\":{\"pressure\":{\"output\":{\"magnitude\":0.0300103,\"unit\":3},\"error\":{\"magnitude\":0.0041932683,\"unit\":7}},\"temperature\":{\"output\":{\"magnitude\":-0.745727,\"unit\":4},\"error\":{\"magnitude\":-0.11576559,\"unit\":4}}}}}},{\"reference\"
